vi "Measurement Logic.vi"(8 "error in":errorcluster, 10 "measure call context in":refnum<class "Measure Call Context.lvclass">, 11 "measurement configuration":T2={"DAQmx Physical Channel"="", "frequency"=1000.0, "amplitude"=1.0, "offset"=0.0, "duration"=1.0} {"duration" format="%#_g s"; "offset" format="%#_g V"; "amplitude" min=0.0 max=10.0 step=1.0 format="%#_g V"; "frequency" min=10.0 max=22000.0 step=1.0 format="%#_4p Hz"}) -> (0 "error out":errorcluster, 2 "measure call context out":refnum<class "Measure Call Context.lvclass">, 3 "measurement results":T1 {"last update" format="%<%x %.3X>T"; "start" format="%<%x %.3X>T"})   [LabVIEW 2022 SP3, in "PureTone Generation.lvlib"]
uses:
  PureTone Generation.lvlib
  Measurement Configuration.ctl
  Measurement Results.ctl
  <vilib>/MeasurementLink/MeasurementLink Measurement Server/Measure Call Context/Measure Call Context.lvclass
  <vilib>/DAQmx/create/channels.llb/DAQmx Create Channel (AO-FuncGen).vi
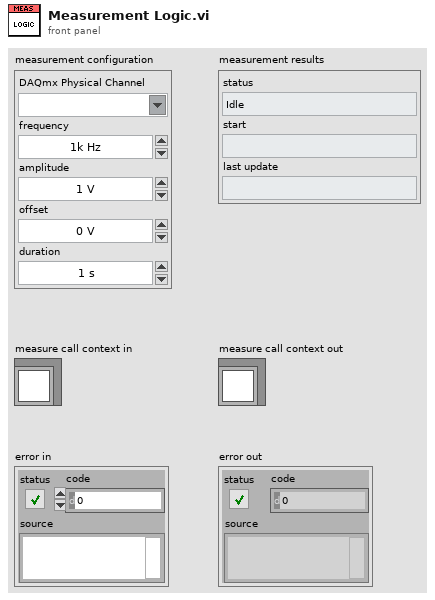
[diagram p1: front panel]
types:
  T1 = typedef "PureTone Generation.lvlib/Measurement Results.ctl" = cluster{"status":enum16{"Idle", "Active", "Error"}, "start":timestamp, "last update":timestamp}
  T2 = typedef "PureTone Generation.lvlib/Measurement Configuration.ctl" = cluster{"DAQmx Physical Channel":tag, "frequency":dbl, "amplitude":dbl, "offset":dbl, "duration":dbl}
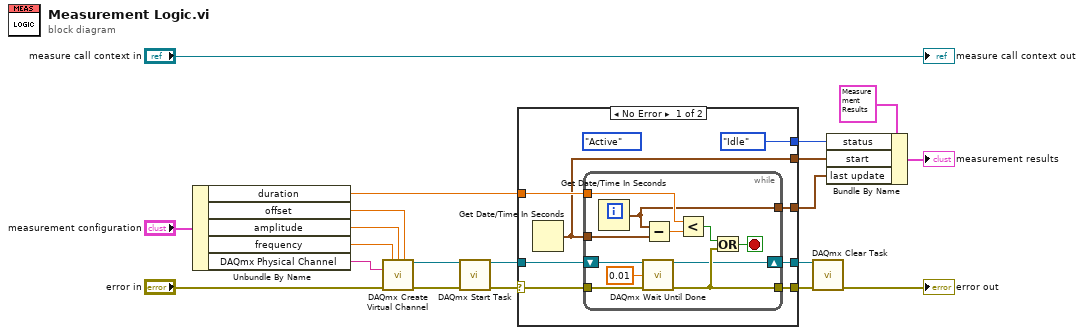
[diagram p0: block diagram]
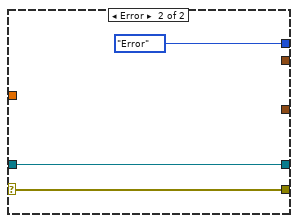
[diagram p2: hidden frame]
diagram:
  n1 = Unbundle By Name("measurement configuration") -> ("duration"=w7:dbl, "offset"=w9:dbl, "amplitude"=w10:dbl, "frequency"=w11:dbl, "DAQmx Physical Channel"=w12:tag)
  n2 = call-poly <vilib>:"DAQmx Create Virtual Channel.vi"("frequency"=w11, "amplitude"=w10, "offset"=w9, "physical channels"=w12, "error in"="error in") -> ("task out"=w19:refnum<k21>, "error out"=w18:errorcluster)  [unwired: 9 in]
  n3 = call <vilib>:"DAQmx Start Task.vi"("task/channels in"=w19, "error in"=w18) -> ("task out"=w17:refnum<k21>, "error out"=w16:errorcluster)  [unwired: 12 in]
  n4 = case shown="No Error" w16 {
    selector: w16 -> [w27 w42]
    tunnel: w17 -> [w28 w41]
    tunnel: [w26 w42] -> w15
    tunnel: [w25 w41] -> w14
    tunnel: w7 -> [w24 _]
    tunnel: [enum16{"Idle", "Active", "Error"}."Idle" ("status") enum16{"Idle", "Active", "Error"}."Error" ("status")] -> w5
    tunnel: [w22 _] -> w2
    tunnel: [w21 _] -> w1
    frame No Error {
      (unwired) enum16{"Idle", "Active", "Error"}."Active" ("status")
      n5 = Get Date/Time In Seconds() -> (seconds since 1Jan1904=w22:timestamp)
      n6 = while {
        tunnel: w27 -> [w36]
        tunnel: [w35] -> w26
        shift-right: [w34] -> w25
        shift-left: w28 -> [w39]
        tunnel: w22 -> [w30]
        tunnel: w24 -> [w33]
        tunnel: [w29] -> w21
        stop <- w37 stop-if-true
        n7 = Get Date/Time In Seconds() -> (seconds since 1Jan1904=w29:timestamp)
        n8 = call <vilib>:"DAQmx Wait Until Done.vi"("task/channels in"=w39, "timeout (sec)"=0.01, "error in"=w36) -> ("task out"=w34:refnum<k21>, "error out"=w35:errorcluster)  [unwired: 11 in]
        n9 = Subtract(x=w29, y=w30) -> (x-y=w32:dbl)
        n10 = Less?(x=w33, y=w32) -> (x < y?=w31:bool)
        n11 = Or(x=w31, y=w35) -> (x .or. y?=w37:bool)
      }
    }
    frame Error {
    }
  }
  n12 = call <vilib>:"DAQmx Clear Task.vi"("task in"=w14, "error in"=w15) -> ("error out"=→"error out":errorcluster)  [unwired: 13 in]
  n13 = Bundle By Name(cluster=T1 {"status"=enum."Idle", "start"=timestamp(0 s since 1904-01-01), "last update"=timestamp(0 s since 1904-01-01)} ("measurement results"), "status"=w5, "start"=w2, "last update"=w1) -> (→"measurement results":T1)
  "measure call context out" <- "measure call context in"
